vi "analysis_images3.vi"() -> ()   [LabVIEW 2019]
uses:
  7e63c831-55bc-40f8-91b0-7870459bb8d8.vi
  <userlib>/_OpenG.lib/array/array.llb/Search 1D Array (DBL)__ogtk.vi
  <vilib>/gmath/NI_Gmath.lvlib
  <vilib>/Analysis/NI_AALBase.lvlib
panel:
  out "Array 2":dbl[](array[numeric])
  out "Array":bool[](array[boolean])
  in  "ilter periods on":dbl format="%#_13g"
  out "Focusing vs periods off filtered":cluster{dbl[], dbl[]}[](graph)
  in  "Update":bool
  in  "stop":bool
  out "array with duplicates removed":dbl[](array[numeric])
  out "Focusing vs periods off":cluster{dbl, "Numeric":dbl}[](graph)
  out "size(s)":i32
  out "CV":dbl
  out "variance":dbl format="%0.2f"
  out "standard deviation":dbl format="%0.2f"
  out "mean":dbl format="%0.2f"
  out "XY Graph 6":cluster{timestamp[], dbl[]}(graph)
  out "element":timestamp
  in  "Repeats":bool
  in  "Controls":bool
  out "Focusing vs periods on":cluster{dbl, "Numeric":dbl}[](graph)
  out "XY Graph 3":cluster{"Best Linear Fit":dbl[], dbl[]}[](graph)
  out "XY Graph 2":cluster{dbl, "Numeric":dbl}[](graph)
  out "XY Graph":cluster{dbl[], "Y":dbl[]}[](graph)
  in  "directory path":path
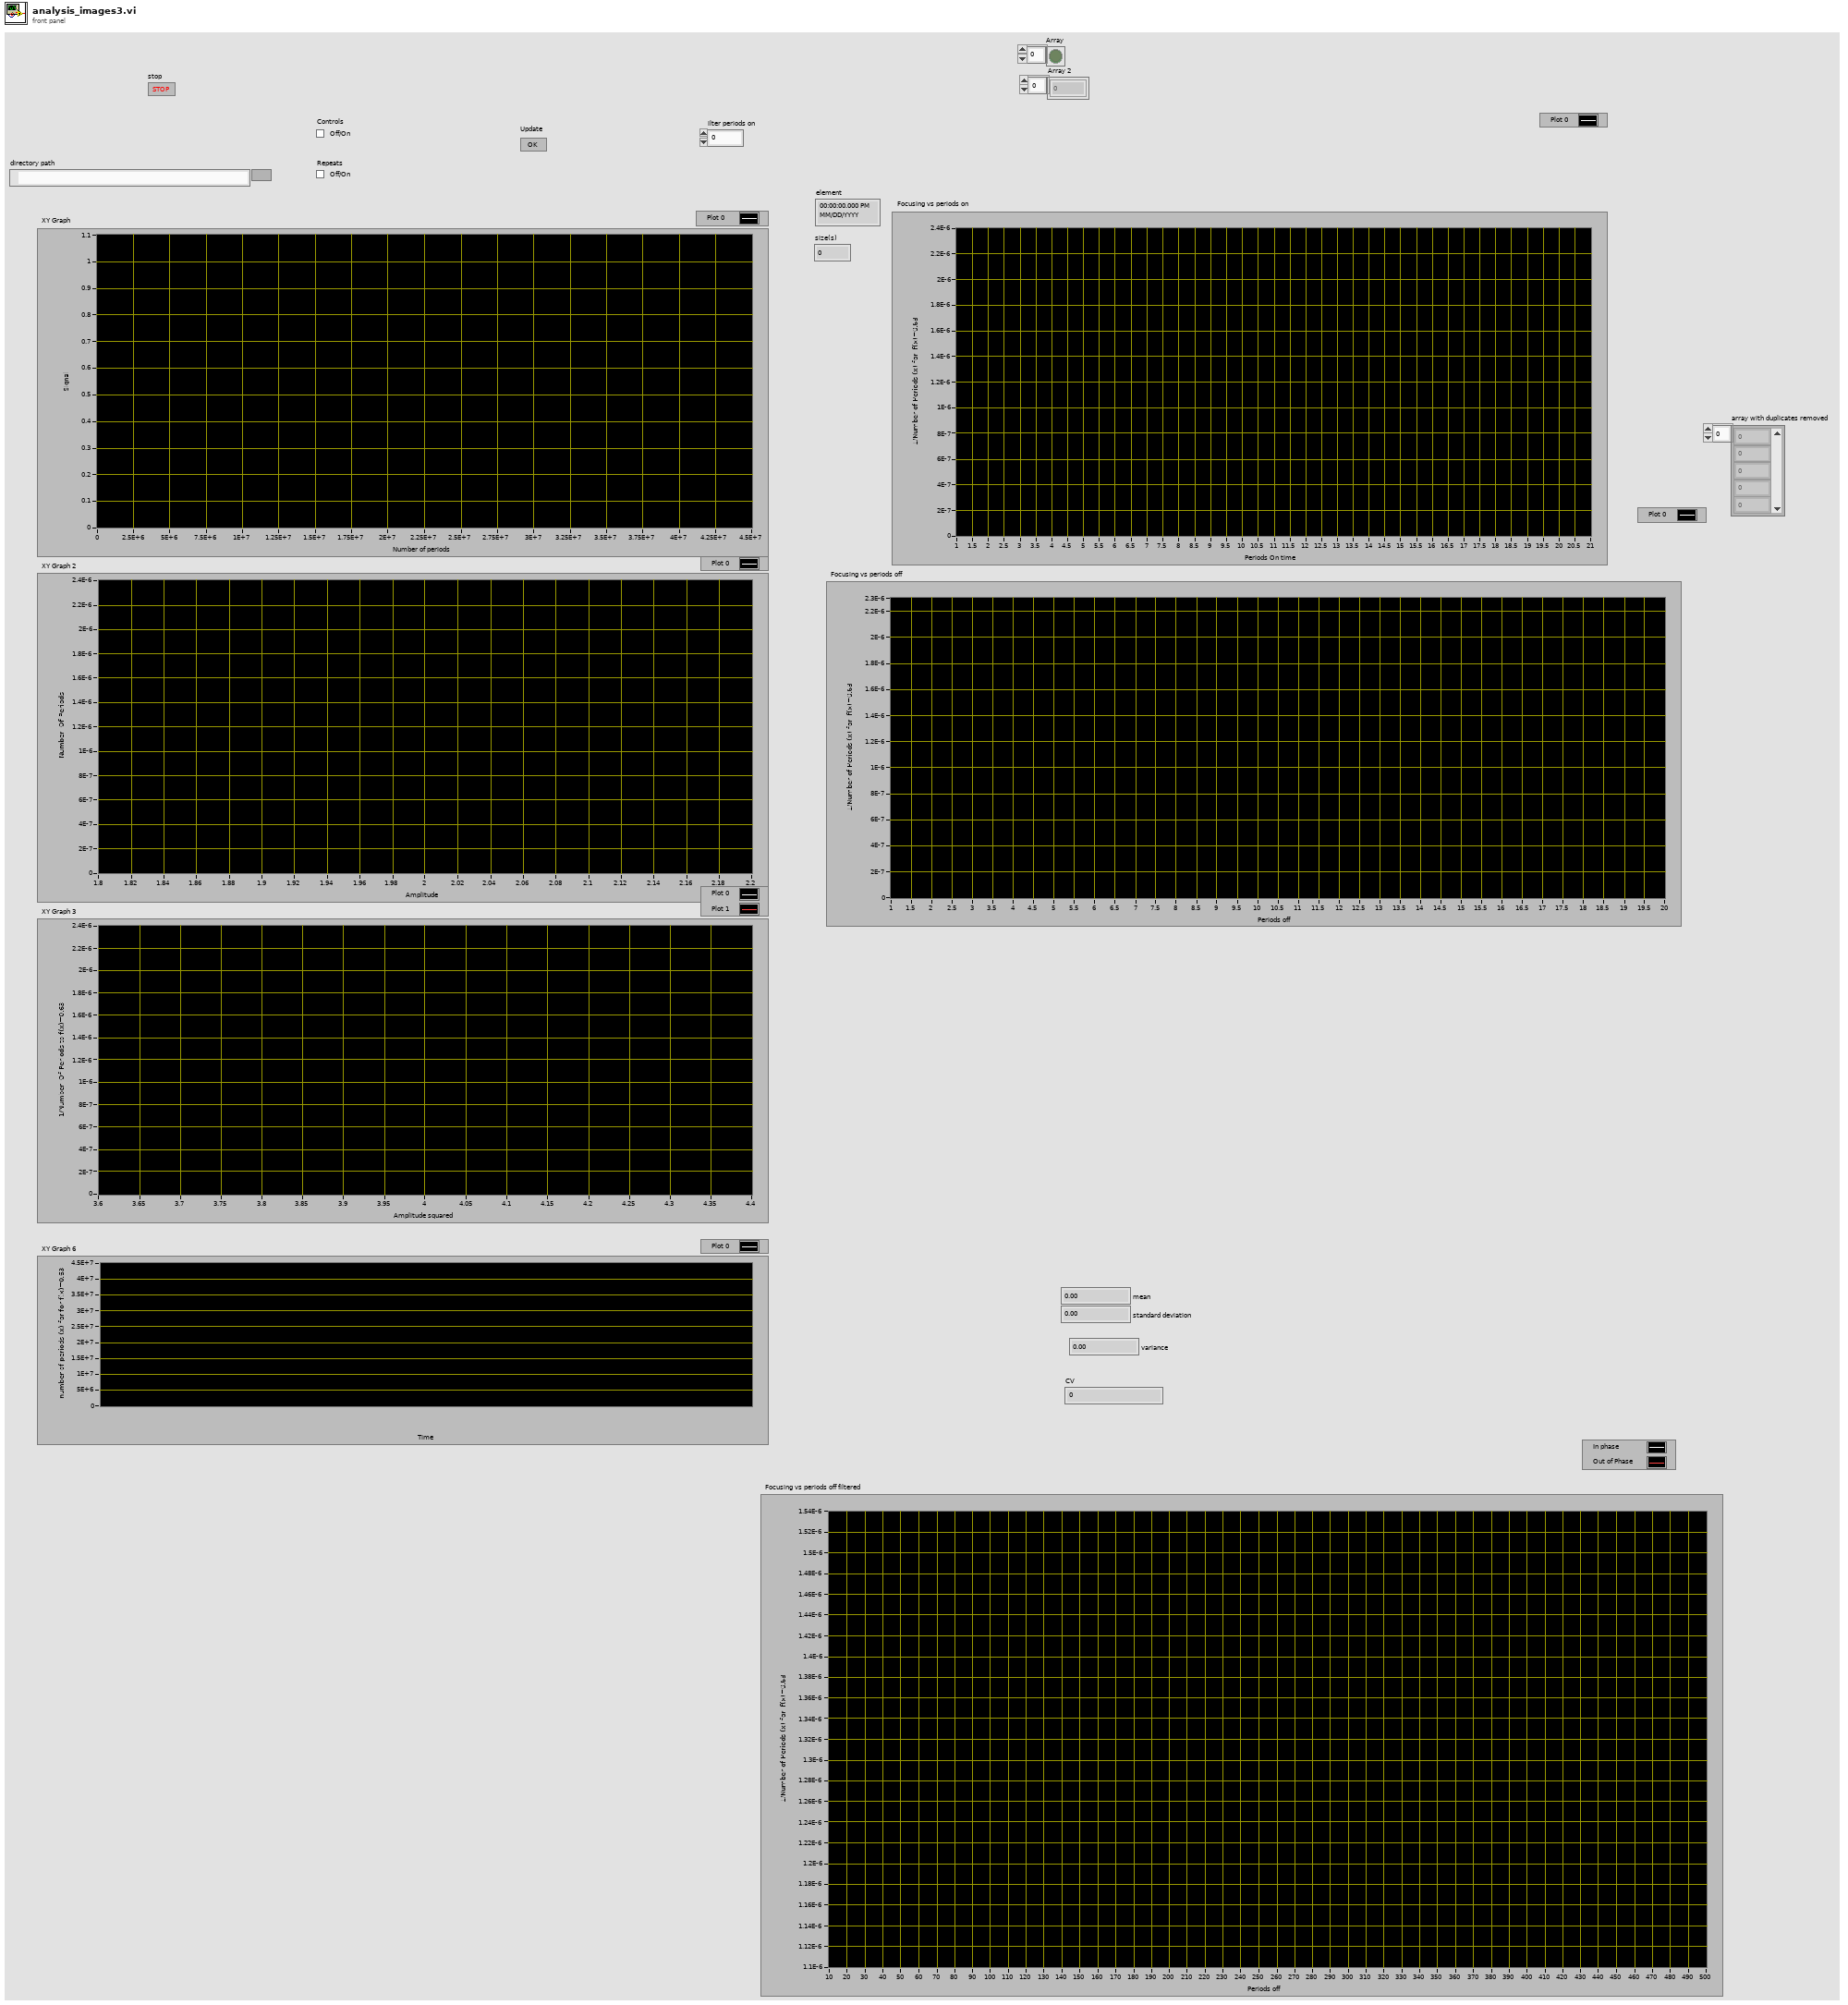
[diagram p1: front panel]
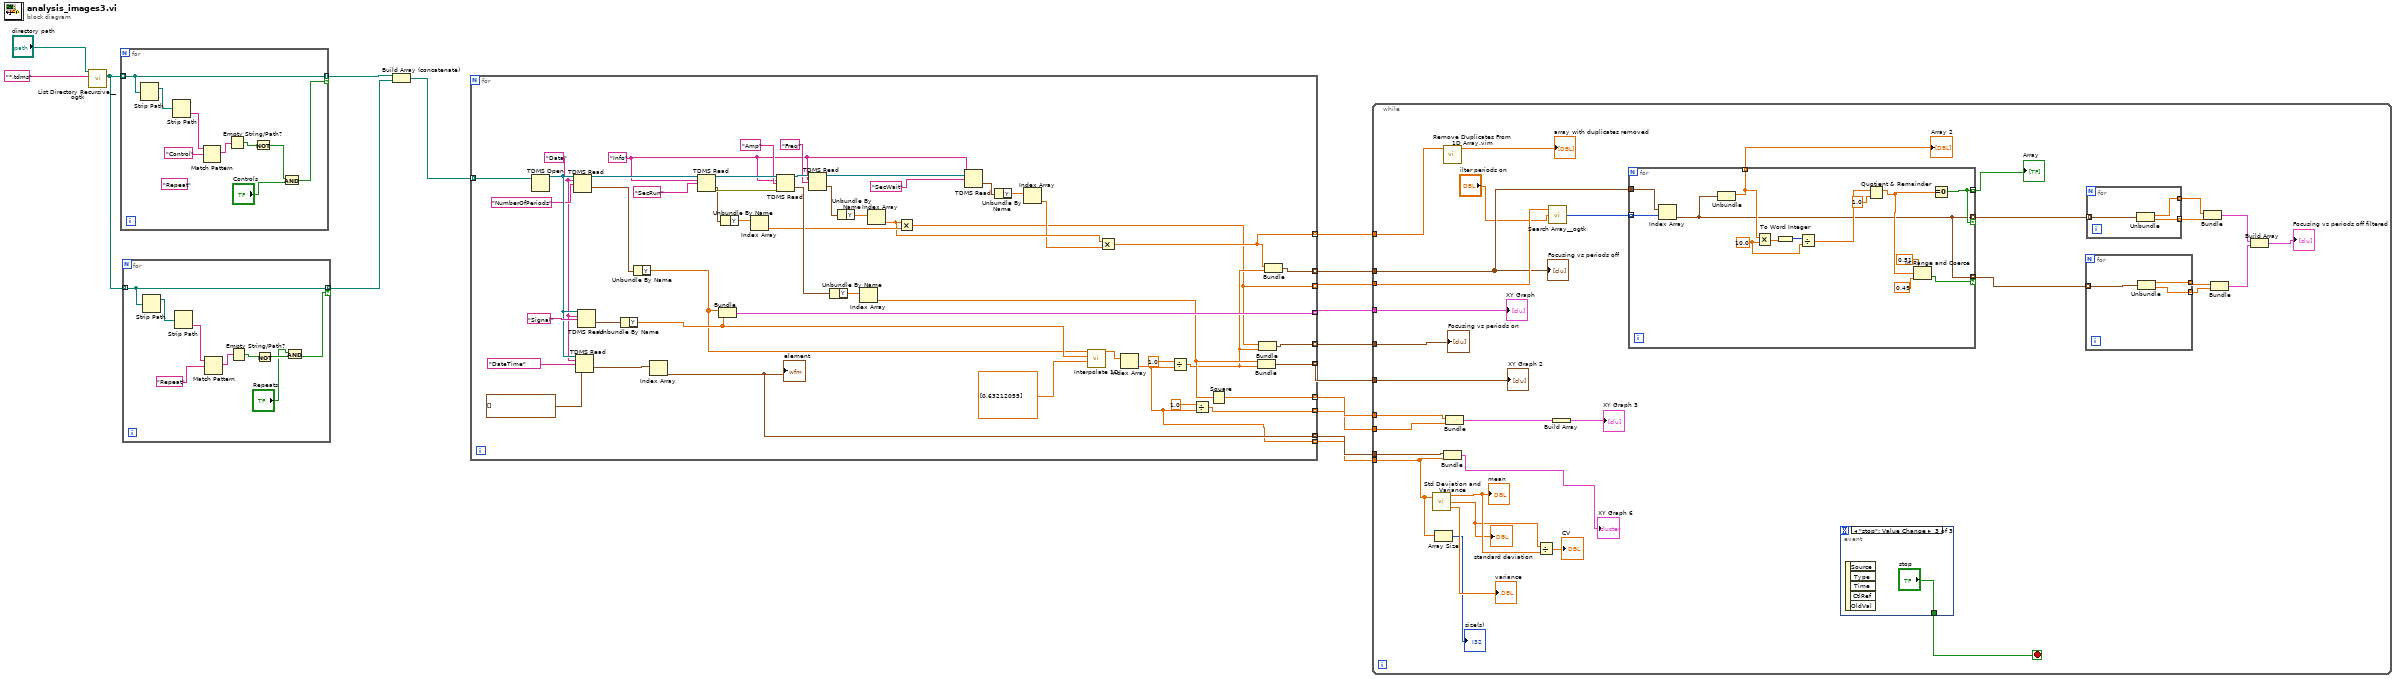
[diagram p0: block diagram]
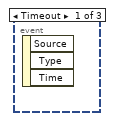
[diagram p2: hidden frame]
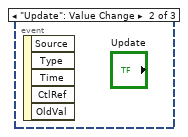
[diagram p3: hidden frame]
diagram:
  n1 = call <userlib>:"List Directory Recursive__ogtk.vi"("pattern"="*.tdms", "Path"="directory path") -> ("file paths"=w10:path[])  [unwired: 6 in, 3 out]
  n2 = for {
    tunnel: w10 -> [w22] mode=indexing
    tunnel: [w22] -> w8 mode=indexing if=w17
    (unwired) "Repeat" ("group name in")
    n3 = Strip Path(path=w22) -> (stripped path=w25:path)  [unwired: 1 out]
    n4 = Strip Path(path=w25) -> (name=w24:string)  [unwired: 1 out]
    n5 = Match Pattern(string=w24, regular expression="Control" ("group name in")) -> (match substring=w23:string)  [unwired: 1 in, 3 out]
    n6 = Empty String/Path?(string/path=w23) -> (empty?=w21:bool)
    n7 = Not(x=w21) -> (.not. x?=w18:bool)
    n8 = And(x=w18, y="Controls") -> (x .and. y?=w17:bool)
  }
  n9 = for {
    tunnel: w10 -> [w31] mode=indexing
    tunnel: [w31] -> w7 mode=indexing if=w27
    n10 = Strip Path(path=w31) -> (stripped path=w34:path)  [unwired: 1 out]
    n11 = Strip Path(path=w34) -> (name=w33:string)  [unwired: 1 out]
    n12 = Match Pattern(string=w33, regular expression="Repeat" ("group name in")) -> (match substring=w32:string)  [unwired: 1 in, 3 out]
    n13 = Empty String/Path?(string/path=w32) -> (empty?=w30:bool)
    n14 = Not(x=w30) -> (.not. x?=w29:bool)
    n15 = And(x="Repeats", y=w29) -> (x .and. y?=w27:bool)
  }
  n16 = Build Array (concatenate)(w8, w7) -> (w9:path[])
  n17 = for {
    tunnel: [w78] -> w14 mode=indexing
    tunnel: [w71] -> w13 mode=indexing
    tunnel: w9 -> [w70] mode=indexing
    tunnel: [w66] -> w12 mode=indexing
    tunnel: [w51] -> w11 mode=indexing
    tunnel: [w59] -> w3 mode=indexing
    tunnel: [w52] -> w6 mode=indexing
    tunnel: [w38] -> w5 mode=indexing
    tunnel: [w40] -> w1 mode=indexing
    tunnel: [w36] -> w4 mode=indexing
    tunnel: [w35] -> w2 mode=indexing
    w45 = "Info" ("group name in")
    w56 = "Data" ("group name in")
    n18 = TDMS Open(11:w70) -> (3:w58:refnum<k34>)  [unwired: 6 in, 1 out]
    n19 = TDMS Read(0:w58, 5:w56, 7:"NumberOfPeriods" ("group name in")) -> (4:w82:refnum<k34>, 10:w83:waveform(dbl))  [unwired: 5 in, 4 out]
    n20 = TDMS Read(0:w58, 5:w56, 7:"DateTime" ("group name in"), 12:timestamp[] []) -> (10:w54:timestamp[])  [unwired: 4 in, 5 out]
    n21 = TDMS Read(0:w58, 5:w56, 7:"Signal" ("group name in")) -> (10:w80:waveform(dbl))  [unwired: 5 in, 5 out]
    n22 = Unbundle By Name(w80) -> ("Y"=w50:dbl[])
    n23 = Unbundle By Name(w83) -> ("Y"=w49:dbl[])
    n24 = Index Array(array=w54) -> (element=w52:timestamp)  [unwired: 1 in]
    "element" <- w52
    n25 = TDMS Read(0:w82, 5:w45, 7:"SecRun" ("group name in")) -> (4:w76:refnum<k34>, 10:w60:waveform(dbl), 15:w75:errorcluster)  [unwired: 5 in, 3 out]
    n26 = Bundle("Y"=w49, "Y"=w50) -> (w78:cluster{"Y":dbl[], "Y":dbl[]})  [unwired: 1 in]
    n27 = Unbundle By Name(w60) -> ("Y"=w61:dbl[])
    n28 = Index Array(array=w61) -> (element=w48:dbl)  [unwired: 1 in]
    n29 = TDMS Read(0:w76, 5:w45, 7:"Amp" ("group name in"), 11:w75) -> (4:w65:refnum<k34>, 10:w73:waveform(dbl))  [unwired: 4 in, 4 out]
    n30 = TDMS Read(0:w65, 5:w45, 7:"Freq" ("group name in")) -> (4:w44:refnum<k34>, 10:w62:waveform(dbl))  [unwired: 5 in, 4 out]
    n31 = Unbundle By Name(w73) -> ("Y"=w72:dbl[])
    n32 = Unbundle By Name(w62) -> ("Y"=w63:dbl[])
    n33 = Index Array(array=w72) -> (element=w68:dbl)  [unwired: 1 in]
    n34 = Index Array(array=w63) -> (element=w42:dbl)  [unwired: 1 in]
    n35 = Multiply(x=w42, y=w48) -> (x*y=w35:dbl)
    n36 = TDMS Read(0:w44, 5:w45, 7:"SecWait" ("group name in")) -> (10:w47:waveform(dbl))  [unwired: 5 in, 5 out]
    n37 = Unbundle By Name(w47) -> ("Y"=w46:dbl[])
    n38 = Index Array(array=w46) -> (element=w41:dbl)  [unwired: 1 in]
    n39 = call <vilib>:"Interpolate 1D.vi"("xi"=dbl[] [0.63212055], "X"=w50, "Y"=w49) -> ("yi"=w69:dbl[])  [unwired: 6 in, 2 out]
    n40 = Multiply(x=w42, y=w41) -> (x*y=w36:dbl)
    n41 = Index Array(array=w69) -> (element=w38:dbl)  [unwired: 1 in]
    n42 = Divide(x=1.0, y=w38) -> (x/y=w37:dbl)
    n43 = Divide(x=1.0, y=w38) -> (x/y=w51:dbl)
    n44 = Square(x=w68) -> (x^2=w66:dbl)
    n45 = Bundle(w68, w37) -> (w71:cluster{dbl, dbl})  [unwired: 1 in]
    n46 = Bundle(w35, w37) -> (w59:cluster{dbl, dbl})  [unwired: 1 in]
    n47 = Bundle(w36, w37) -> (w40:cluster{dbl, dbl})  [unwired: 1 in]
  }
  n48 = while {
    tunnel: w14 -> [w116]
    tunnel: w13 -> [w115]
    tunnel: w12 -> [w114]
    tunnel: w11 -> [w113]
    tunnel: w6 -> [w110]
    tunnel: w5 -> [w104]
    tunnel: w4 -> [w102]
    tunnel: w3 -> [w98]
    tunnel: w2 -> [w100]
    tunnel: w1 -> [w97]
    stop <- w84 stop-if-true
    n49 = call <vilib>:"Std Deviation and Variance.vi"("X"=w104) -> ("mean"=w106:dbl, "standard deviation"=w105:dbl, "variance"=→"variance":dbl)  [unwired: 1 in]
    "mean" <- w106
    "standard deviation" <- w105
    n50 = Array Size(array=w104) -> (size(s)=→"size(s)":i32)
    n51 = call "Remove Duplicates From 1D Array.vim"("array"=w102) -> ("array with duplicates removed"=→"array with duplicates removed":dbl[])  [unwired: 10 in]
    n52 = Bundle(w110, w104) -> (→"XY Graph 6":cluster{timestamp[], dbl[]})  [unwired: 1 in]
    n53 = Bundle(w114, w113) -> (w112:cluster{dbl[], dbl[]})  [unwired: 1 in]
    n54 = Divide(x=w105, y=w106) -> (x/y=→"CV":dbl)
    n55 = call-poly <userlib>:"Search Array__ogtk.vi"("Array"=w100, "Element Data"="ilter periods on") -> ("Indices of Elements"=w99:i32[])  [unwired: 7 in]
    n56 = Build Array(w112) -> (→"XY Graph 3":cluster{dbl[], dbl[]}[])
    n57 = for {
      tunnel: w99 -> [w136] mode=indexing
      tunnel: w97 -> [w135]
      tunnel: [w124] -> w92 mode=indexing if=w125
      tunnel: [w125] -> w95 mode=indexing
      tunnel: [w127] -> w94 mode=indexing
      tunnel: [w124] -> w93 mode=indexing if=w123
      w129 = 10.0 ("y")
      n58 = Index Array(array=w135, index=w136) -> (element=w124:cluster{dbl, dbl})
      n59 = Unbundle(w124) -> (w127:dbl)  [unwired: 1 out]
      n60 = Multiply(x=w127, y=w129) -> (x*y=w130:dbl)
      n61 = To Word Integer(number=w130) -> (16bit integer=w128:i16)
      n62 = Divide(x=w128, y=w129) -> (x/y=w126:dbl)
      n63 = Quotient & Remainder(x=w126, y=1.0) -> (x-y*floor(x/y)=w131:dbl)  [unwired: 1 out]
      n64 = In Range and Coerce(upper limit=0.51, x=w131, lower limit=0.49) -> (In Range?=w123:bool)  [unwired: 1 out]
      n65 = Equal To 0?(x=w131) -> (x = 0?=w125:bool)
    }
    "Array" <- w95
    "Array 2" <- w94
    n66 = event shown="[2] \"stop\": Value Change" {
      selector: _ -> [_ _ _]
      dyn-events: _ -> [_ _ _]
      timeout: _ -> [_ _ _]
      tunnel: [_ _ "stop"] -> w84
      event Timeout {
        n67 = event-data() -> ()  [unwired: 1 in, 3 out]
      }
      event "Update": Value Change {
        n68 = event-data() -> ()  [unwired: 1 in, 5 out]
      }
      event "stop": Value Change {
        n69 = event-data() -> ()  [unwired: 1 in, 5 out]
      }
    }
    n70 = for {
      tunnel: w93 -> [w119] mode=indexing
      tunnel: [w118] -> w88 mode=indexing
      tunnel: [w117] -> w89 mode=indexing
      n71 = Unbundle(w119) -> (w118:dbl, w117:dbl)
    }
    n72 = for {
      tunnel: w92 -> [w122] mode=indexing
      tunnel: [w121] -> w90 mode=indexing
      tunnel: [w120] -> w91 mode=indexing
      n73 = Unbundle(w122) -> (w121:dbl, w120:dbl)
    }
    n74 = Bundle(w90, w91) -> (w86:cluster{dbl[], dbl[]})  [unwired: 1 in]
    n75 = Bundle(w88, w89) -> (w87:cluster{dbl[], dbl[]})  [unwired: 1 in]
    n76 = Build Array(w86, w87) -> (→"Focusing vs periods off filtered":cluster{dbl[], dbl[]}[])
    "XY Graph" <- w116
    "XY Graph 2" <- w115
    "Focusing vs periods on" <- w98
    "Focusing vs periods off" <- w97
  }
